vi "Send Transfer Group.vi"(7 "Command":T1=enum."Rx", 8 "error in (no error)":errorcluster, 9 "Transfer Group iteration":u64, 10 "Transfer Group ID":i32, 11 "Plugin Interface in":refnum<class "Plugin Interface.lvclass">) -> (0 "error out":errorcluster, 3 "Plugin Interface out":refnum<class "Plugin Interface.lvclass">)   [LabVIEW 2017, in "DSF Core.lvlib" / "Plugin Interface.lvclass"]
uses:
  Plugin Interface.lvclass
  C:/Users/Admin/Desktop/Data Sharing Framework/Source/Core/Engine/Classes/Interfaces/Interface/Interface.lvclass
  Command.ctl
  Command Data.ctl
  Command Parameters.ctl
  Interface/Interface.lvclass/Interface.ctl
  Write Plugin Command.vi
  Interface/Write Command.vi
  Interface/Write RT FIFO.vi
  Interface/Errors.vi
  Dispatcher/Command Timeout.vi
  Class Name.vi
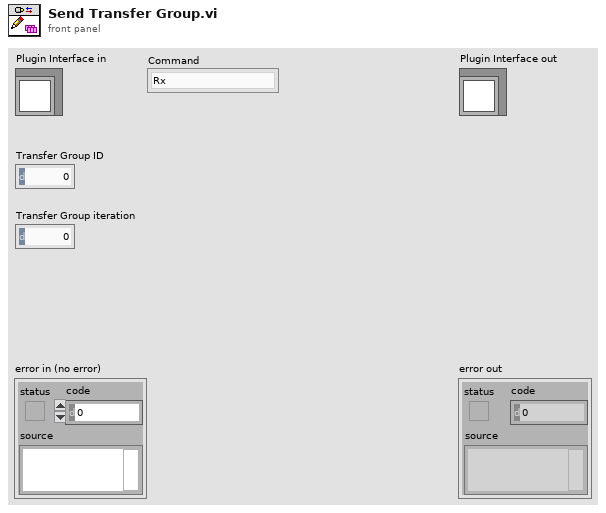
[diagram p1: front panel]
types:
  T1 = typedef "DSF Core.lvlib/Plugin Interface.lvclass/Command.ctl" = enum8{"Set Inline Buffer", "Rx", "Tx", "Shutdown"}
  T2 = cluster{"Transfer Group ID":i32, "unused 0":i32, "Transfer Group iteration":u64}
  T3 = typedef "DSF Core.lvlib/Plugin Interface.lvclass/Command Parameters.ctl" = cluster{"arg1":u64, "arg2":u64}
  T4 = typedef "DSF Core.lvlib/Plugin Interface.lvclass/Command Data.ctl" = cluster{"Command":T1, "Parameters":T3}
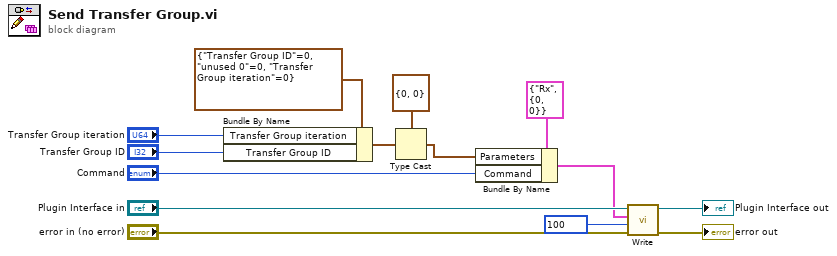
[diagram p0: block diagram]
diagram:
  n1 = Bundle By Name(cluster=T2 {"Transfer Group ID"=0, "unused 0"=0, "Transfer Group iteration"=0}, "Transfer Group iteration"="Transfer Group iteration", "Transfer Group ID"="Transfer Group ID") -> (w10:T2)
  n2 = Type Cast(type=T3 {"arg1"=0, "arg2"=0} ("Command Parameters"), x=w10) -> (*(type *) &x=w12:T3)
  n3 = Bundle By Name(cluster=T4 {"Command"=enum."Rx", "Parameters"={"arg1"=0, "arg2"=0}} ("command"), "Parameters"=w12, "Command"="Command") -> (w1:T4)
  n4 = call-poly "Write.vi"("error in (no error)"="error in (no error)", "timeout in ms (0)"=100, "command"=w1, "Plugin Interface in"="Plugin Interface in") -> ("error out"=→"error out":errorcluster, "Plugin Interface out"=→"Plugin Interface out":refnum<class "Plugin Interface.lvclass">)  [unwired: 6 in]
